vi "Deadband.vi"(9 "Deadband":dbl, 10 "Before Deadband":dbl, 11 "Expand Range":bool) -> (2 "After Deadband":dbl)   [LabVIEW 2014, in "Joystick.lvlib"]
uses:
  Joystick.lvlib
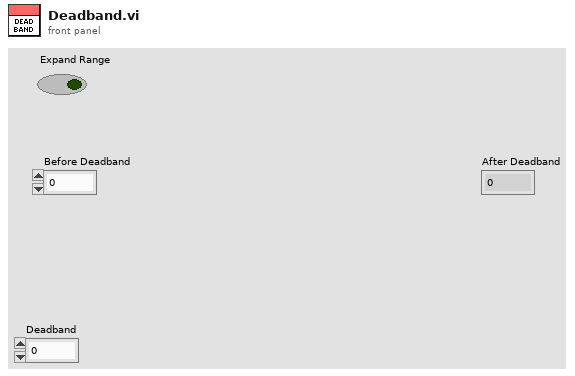
[diagram p1: front panel]
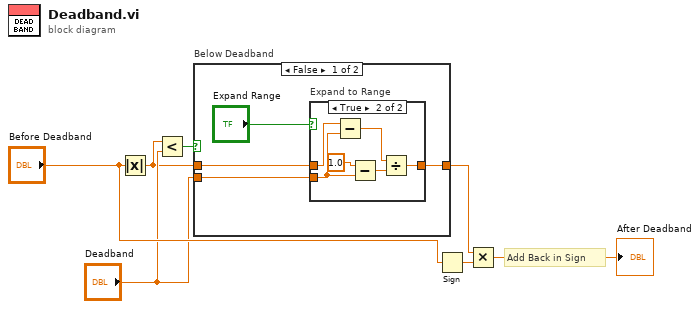
[diagram p0: block diagram]
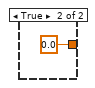
[diagram p3: hidden frame]
diagram:
  # "Add Back in Sign"
  n1 = Absolute Value(x="Before Deadband") -> (abs(x)=w1:dbl)
  n2 = Less?(x=w1, y="Deadband") -> (x < y?=w7:bool)
  n3 = case "Below Deadband" shown="False" w7 {
    tunnel: w1 -> [w10 _]
    tunnel: [w9 0.0 ("Before Deadband")] -> w6
    tunnel: "Deadband" -> [w8 _]
    frame False {
      n4 = case "Expand to Range" shown="True" "Expand Range" {
        tunnel: w10 -> [w12 w18]
        tunnel: [w12 w13] -> w9
        tunnel: w8 -> [_ w15]
        frame False {
        }
        frame True {
          n5 = Subtract(x=w18, y=w15) -> (x-y=w17:dbl)
          n6 = Subtract(x=1.0, y=w15) -> (x-y=w14:dbl)
          n7 = Divide(x=w17, y=w14) -> (x/y=w13:dbl)
        }
      }
    }
    frame True {
    }
  }
  n8 = Sign(1:"Before Deadband") -> (0:w3:dbl)
  n9 = Multiply(x=w6, y=w3) -> (x*y=→"After Deadband":dbl)
